vi "GetText.vi"(8 "error in":errorcluster, 11 "RTResourceUtilitzation editor node in":refnum<class "RTResourceUtilitzation editor node.lvclass">) -> (0 "error out":errorcluster, 1 "additional text":string, 2 "text":string, 3 "RTResourceUtilitzation editor node out":refnum<class "RTResourceUtilitzation editor node.lvclass">, 4 "glyph":string)   [LabVIEW 2014, in "RTResourceUtilitzation editor node.lvclass"]
uses:
  RTResourceUtilitzation editor node.lvclass
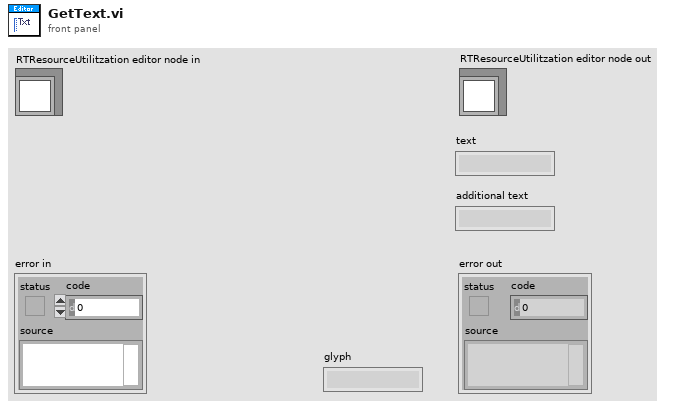
[diagram p1: front panel]
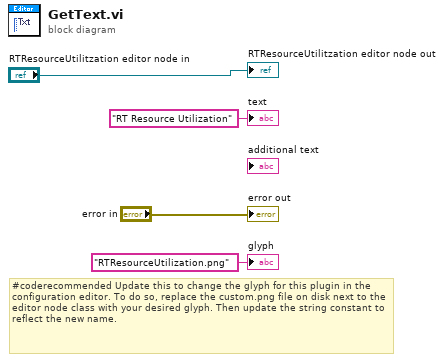
[diagram p0: block diagram]
diagram:
  # "#coderecommended Update this to change the glyph for this plugin in the configuration editor. To do so, replace the custom.png file on disk next to the editor node class with your desired glyph. Then update the string constant to reflect the new name."
  "error out" <- "error in"
  "RTResourceUtilitzation editor node out" <- "RTResourceUtilitzation editor node in"
  "text" <- "RT Resource Utilization" ("text")
  "glyph" <- "RTResourceUtilization.png" ("glyph")
